vi "Write TestSteps.vi"(8 "error in (no error)":errorcluster, 10 "TestSteps":T1(array[cluster]), 11 "TestSeqClass in":refnum<class "TestSeqClass.lvclass">) -> (0 "error out":errorcluster, 3 "TestSeqClass out":refnum<class "TestSeqClass.lvclass">)   [LabVIEW 2019, in "TestSeqClass.lvclass"]
uses:
  TestSeqClass.lvclass
  TestSeqClass.lvclass/TestSeqClass.ctl
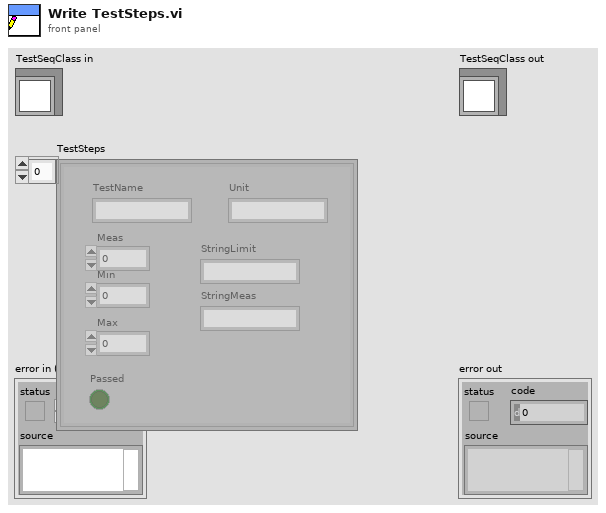
[diagram p1: front panel]
types:
  T1 = cluster{"TestName":string, "Meas":dbl, "Min ":dbl, "Max":dbl, "Passed":bool, "StringLimit":string, "StringMeas":string, "Unit":string}[]
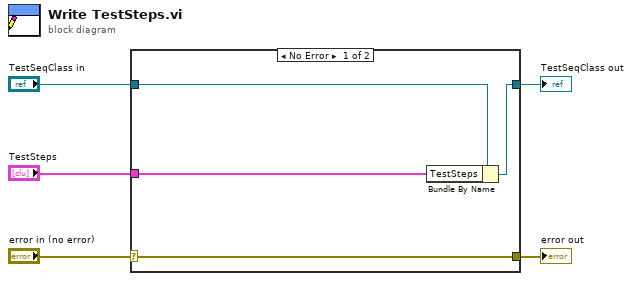
[diagram p0: block diagram]
diagram:
  n1 = case shown="No Error" "error in (no error)" {
    selector: "error in (no error)" -> [w9 w10]
    tunnel: [w9 w10] -> w4
    tunnel: [w7 w11] -> w2
    tunnel: "TestSeqClass in" -> [w8 w11]
    tunnel: "TestSteps" -> [w6 _]
    frame No Error {
      n2 = Bundle By Name(cluster=w8, "TestSteps"=w6) -> (w7:refnum<class "TestSeqClass.lvclass">)
    }
    frame Error {
    }
  }
  "error out" <- w4
  "TestSeqClass out" <- w2
